vi "虚拟放射源数据USB读取（单个数据）.vi"() -> ()   [LabVIEW 2013]
panel:
  in  "信号源":u16(ring) items=["幅度随机数", "初始时间随机数", "最终时间随机数"]
  in  "仪器使能":bool
  in  "数据输出":u16(ring) items=["USB", "DAC"]
  in  "停止":bool
  out "随机数":u16
  out "波形图":i32[](graph)
  out "虚拟放射源VISA":string
  out "数组":i32[](array[numeric])
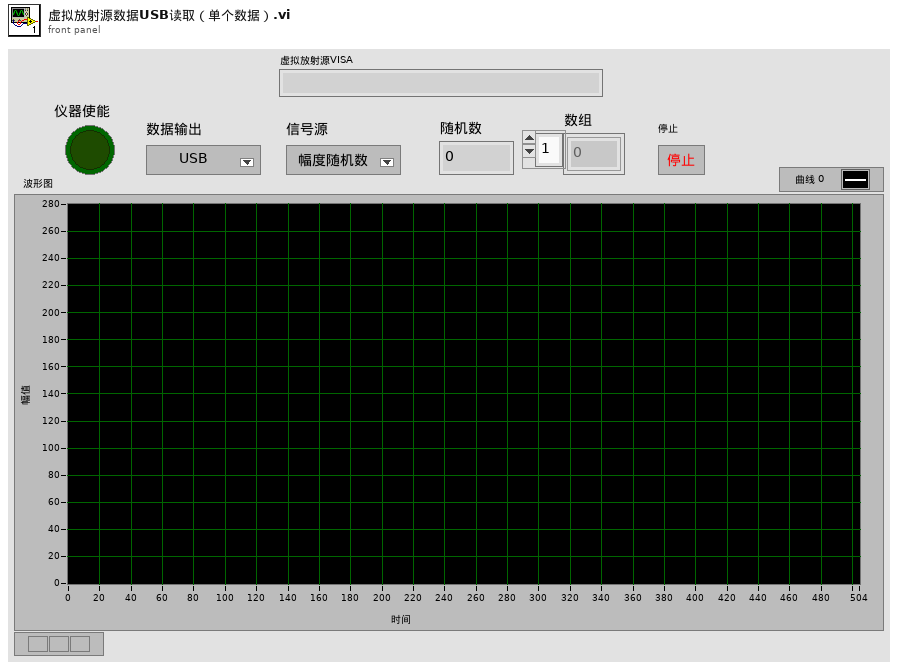
[diagram p1: front panel]
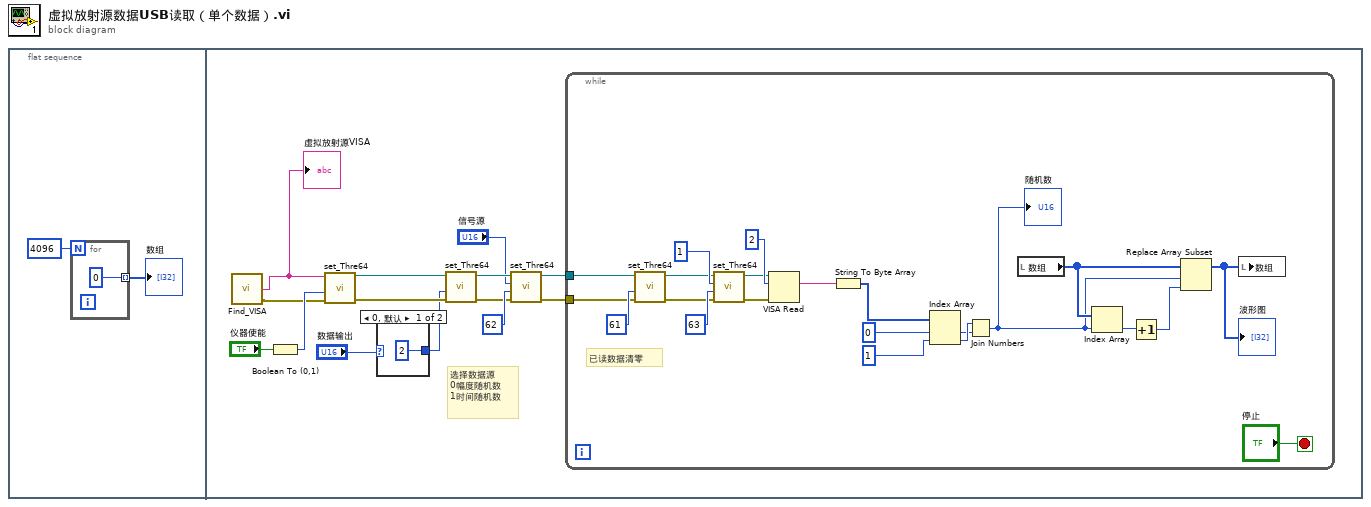
[diagram p0: block diagram]
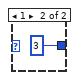
[diagram p2: hidden frame]
diagram:
  n1 = flat-sequence {
    frame #0 {
      n2 = for {
        N: 4096 -> [_]
        tunnel: [0] -> w1 mode=indexing
      }
      "数组" <- w1
    }
    frame #1 {
      # "选择数据源\n0幅度随机数\n1时间随机数"
      n3 = call "Find_VISA.vi"() -> ("错误输出"=w6:errorcluster, "虚拟放射源VISA"=w5:string)  [unwired: 3 in, 1 out]
      "虚拟放射源VISA" <- w5
      n4 = Boolean To (0,1)(Boolean="仪器使能") -> (0, 1=w16:i16)
      n5 = call "set_Thre64.vi"("错误输入（无错误）"=w6, "命令"=w16, "VISA资源名称"=w5) -> ("错误输出"=w14:errorcluster, "VISA资源名称输出"=w15:refnum<visa-resource-name>)  [unwired: 7 in]
      n6 = case shown="0, 默认" "数据输出" {
        tunnel: [2 3] -> w12
        frame 0, Default {
        }
        frame 1 {
        }
      }
      n7 = call "set_Thre64.vi"("错误输入（无错误）"=w14, "命令"=w12, "VISA资源名称"=w15) -> ("错误输出"=w9:errorcluster, "VISA资源名称输出"=w10:refnum<visa-resource-name>)  [unwired: 7 in]
      n8 = call "set_Thre64.vi"("错误输入（无错误）"=w9, "命令"=u8 62, "数字"="信号源", "VISA资源名称"=w10) -> ("错误输出"=w7:errorcluster, "VISA资源名称输出"=w8:refnum<visa-resource-name>)  [unwired: 6 in]
      n9 = while {
        tunnel: w8 -> [w31]
        tunnel: w7 -> [w30]
        stop <- "停止" stop-if-true
        # "已读数据清零"
        n10 = call "set_Thre64.vi"("错误输入（无错误）"=w30, "命令"=u8 61, "VISA资源名称"=w31) -> ("错误输出"=w28:errorcluster, "VISA资源名称输出"=w29:refnum<visa-resource-name>)  [unwired: 7 in]
        n11 = call "set_Thre64.vi"("错误输入（无错误）"=w28, "命令"=u8 63, "数字"=u16 1, "VISA资源名称"=w29) -> ("错误输出"=w36:errorcluster, "VISA资源名称输出"=w35:refnum<visa-resource-name>)  [unwired: 6 in]
        n12 = VISA Read(VISA resource name=w35, byte count=u32 2 ("字节总数"), error in (no error)=w36) -> (read buffer=w33:string)  [unwired: 3 out]
        n13 = String To Byte Array(string=w33) -> (unsigned byte array=w25:u8[])
        n14 = Index Array(array=w25, index #1=0 ("x"), index #2=1 ("x")) -> (element #1=w26:u8, element #2=w27:u8)
        n15 = Join Numbers(hi=w27, lo=w26) -> ((hi.lo)=w21:u16)
        "随机数" <- w21
        n16 = local read "数组"() -> (w23:i32[])
        n17 = Index Array(array=w23, index=w21) -> (element=w24:i32)
        n18 = Increment(x=w24) -> (x+1=w22:i32)
        n19 = Replace Array Subset(array=w23, new element=w22, index=w21) -> (w20:i32[])
        "波形图" <- w20
        n20 = local write "数组"(w20) -> ()
      }
    }
  }
